vi "RomiSim_WriteSensors.vi"(10 "Diff Drive Train Sim":T8 {"m_Motor"."Jr_KgM2" format="%13.5p"; "m_Motor"."L_H" format="%13.5p"; "m_Motor"."Kt_NMPerAmp" format="%13.5p"; "m_Motor"."KvINV_RadPerSecPerVolt" format="%13.5p"; "m_Motor"."R_Ohms" format="%13.5p"; "m_Motor"."FreeSpeed_RadPerSec" format="%13.5p"; "m_Motor"."FreeCurrent_Amps" format="%13.5p"; "m_Motor"."StallCurrent_Amps" format="%13.5p"; "m_Motor"."StallTorque_NM" format="%13.5p"; "m_Motor"."nominalVoltage_Volts" format="%13.5p"}, 11 "Counts/Feet":dbl) -> (0 "Right Speed Ft/Sec":dbl, 1 "Right Encoder":T6, 2 "Left Speed Ft/Sec":dbl, 3 "Left Encoder":T6, 4 "Robot Pose":T3 {"ROTATION"."SIN" format="%13.4f"; "ROTATION"."COS" format="%13.4f"; "ROTATION"."VALUE" format="%13.4f"; "TRANSLATION"."Y" format="%14.3f"; "TRANSLATION"."X" format="%14.3f"}, 5 "Gyro Deg":dbl, 7 "Gyro":T1)   [LabVIEW 2019]
uses:
  <vilib>/Rock Robotics/WPI/ThirdParty/JAS_Junk/TrajLib/TypeDef/DIFF_DRIVE_TRAIN_SIM.ctl
  <vilib>/Rock Robotics/WPI/ThirdParty/JAS_Junk/TrajLib/TypeDef/LINEAR_SYSTEM.ctl
  <vilib>/Analysis/Matrix/Datatypes/RealMatrix.ctl
  <vilib>/Rock Robotics/WPI/ThirdParty/JAS_Junk/TrajLib/TypeDef/DCMOTOR.CTL
  <vilib>/Rock Robotics/WPI/Simulation/Protocol/Devices/Encoder/Encoder proto.ctl
  <vilib>/Rock Robotics/WPI/Simulation/Protocol/Devices/Encoder/Encoder data protoo.ctl
  <vilib>/Rock Robotics/WPI/ThirdParty/JAS_Junk/TrajLib/TypeDef/POSE2D.ctl
  <vilib>/Rock Robotics/WPI/ThirdParty/JAS_Junk/TrajLib/TypeDef/TRANSLATION2D.ctl
  <vilib>/Rock Robotics/WPI/ThirdParty/JAS_Junk/TrajLib/TypeDef/ROTATION2D.ctl
  <vilib>/Rock Robotics/WPI/Simulation/Protocol/Devices/Gyro/Gyro proto.ctl
  <vilib>/Rock Robotics/WPI/Simulation/Protocol/Devices/Gyro/Gyro Data proto.ctl
  <vilib>/Rock Robotics/WPI/Simulation/Protocol/Devices/Encoder/Encoder Update Ops.ctl
  <vilib>/Rock Robotics/SystemInterfaces/Encoder/FPGA_EncoderIdx.ctl
  <vilib>/Rock Robotics/WPI/Simulation/Protocol/Devices/Gyro/Gyro Update Ops.ctl
  <vilib>/Rock Robotics/WPI/ThirdParty/JAS_Junk/TrajLib/Trajectory_Library.lvlib
  <vilib>/Analysis/Matrix/NI_Matrix.lvlib
panel:
  # "<States, 1>"
  # "<Outputs, 1>"
  # "<Inputs, 1>"
  # "<Outputs, 1>"
  # "<States,States>"
  # "<States,Inputs>"
  # "<Outputs,States>"
  # "<Outputs,Inputs>"
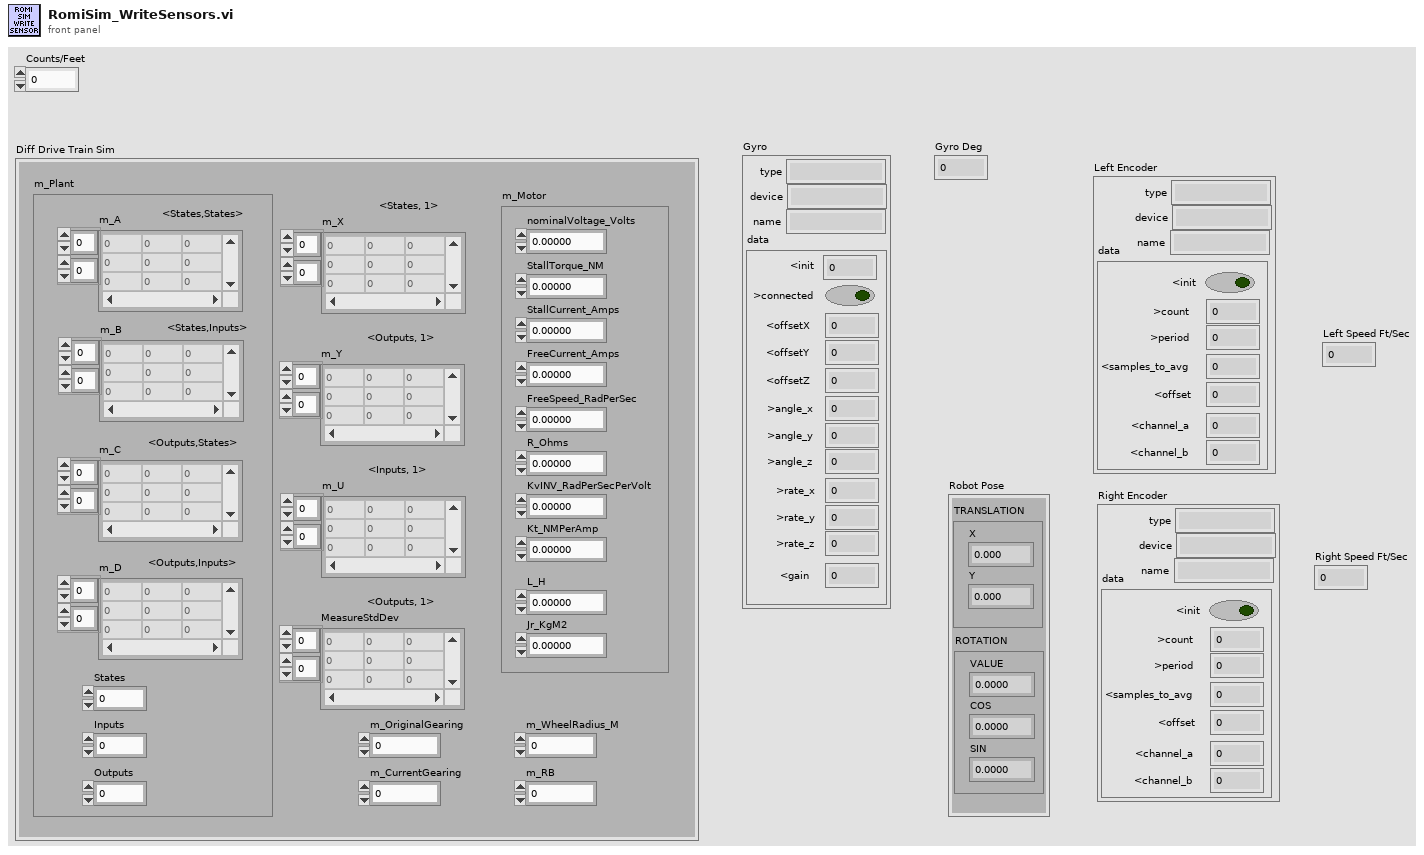
[diagram p1: front panel]
types:
  T1 = typedef "Gyro proto.ctl" = cluster{"type":string, "device":string, "name":string, "data":T2}
  T2 = typedef "Gyro Data proto.ctl" = cluster{"<init":i32, ">connected":bool, "<offsetX":dbl, "<offsetY":dbl, "<offsetZ":dbl, ">angle_x":dbl, ">angle_y":dbl, ">angle_z":dbl, ">rate_x":dbl, ">rate_y":dbl, ">rate_z":dbl, "<gain":dbl}
  T3 = typedef "Trajectory_Library.lvlib/POSE2D.ctl" = cluster{"TRANSLATION":T4, "ROTATION":T5}
  T4 = typedef "Trajectory_Library.lvlib/TRANSLATION2D.ctl" = cluster{"X":dbl, "Y":dbl}
  T5 = typedef "Trajectory_Library.lvlib/ROTATION2D.ctl" = cluster{"VALUE":dbl, "COS":dbl, "SIN":dbl}
  T6 = typedef "Encoder proto.ctl" = cluster{"type":string, "device":string, "name":string, "data":T7}
  T7 = typedef "Encoder data protoo.ctl" = cluster{"<init":bool, ">count":dbl, ">period":dbl, "<samples_to_avg":i32, "<offset":dbl, "<channel_a":i32, "<channel_b":i32}
  T8 = typedef "Trajectory_Library.lvlib/DIFF_DRIVE_TRAIN_SIM.ctl" = cluster{"m_Plant":T9, "m_X":T10, "m_Y":T10, "m_U":T10, "MeasureStdDev":T10, "m_Motor":T11, "m_OriginalGearing":dbl, "m_CurrentGearing":dbl, "m_WheelRadius_M":dbl, "m_RB":dbl}
  T9 = typedef "Trajectory_Library.lvlib/LINEAR_SYSTEM.ctl" = cluster{"m_A":T10, "m_B":T10, "m_C":T10, "m_D":T10, "States":i32, "Inputs":i32, "Outputs":i32}
  T10 = typedef "NI_Matrix.lvlib/RealMatrix.ctl" = dbl[][]
  T11 = typedef "Trajectory_Library.lvlib/DCMOTOR.CTL" = cluster{"nominalVoltage_Volts":dbl, "StallTorque_NM":dbl, "StallCurrent_Amps":dbl, "FreeCurrent_Amps":dbl, "FreeSpeed_RadPerSec":dbl, "R_Ohms":dbl, "KvINV_RadPerSecPerVolt":dbl, "Kt_NMPerAmp":dbl, "L_H":dbl, "Jr_KgM2":dbl}
  T12 = typedef "Gyro Update Ops.ctl" = enum16{"get", "delete", "JSON update", "set  name", "transmit initial", "reset", "set init", "set offsetX", "set offsetY", "set offsetZ", "set gain", "set angle X", "set angle Y", "set angle Z", "set rate X", "set rate Y", "set rate Z"}
  T13 = typedef "Encoder Update Ops.ctl" = enum16{"set init", "set count", "set period", "set reset", "set samples_to_avg", "get", "delete", "JSON update", "set name", "transmit initial", "reset", "set channel_a", "set channel_b"}
  T14 = typedef "FPGA_EncoderIdx.ctl" = enum8{"Enc 0", "Enc 1", "Enc 2", "Enc 3", "Enc 4", "Enc 5", "Enc 6", "Enc 7", "Invalid"}
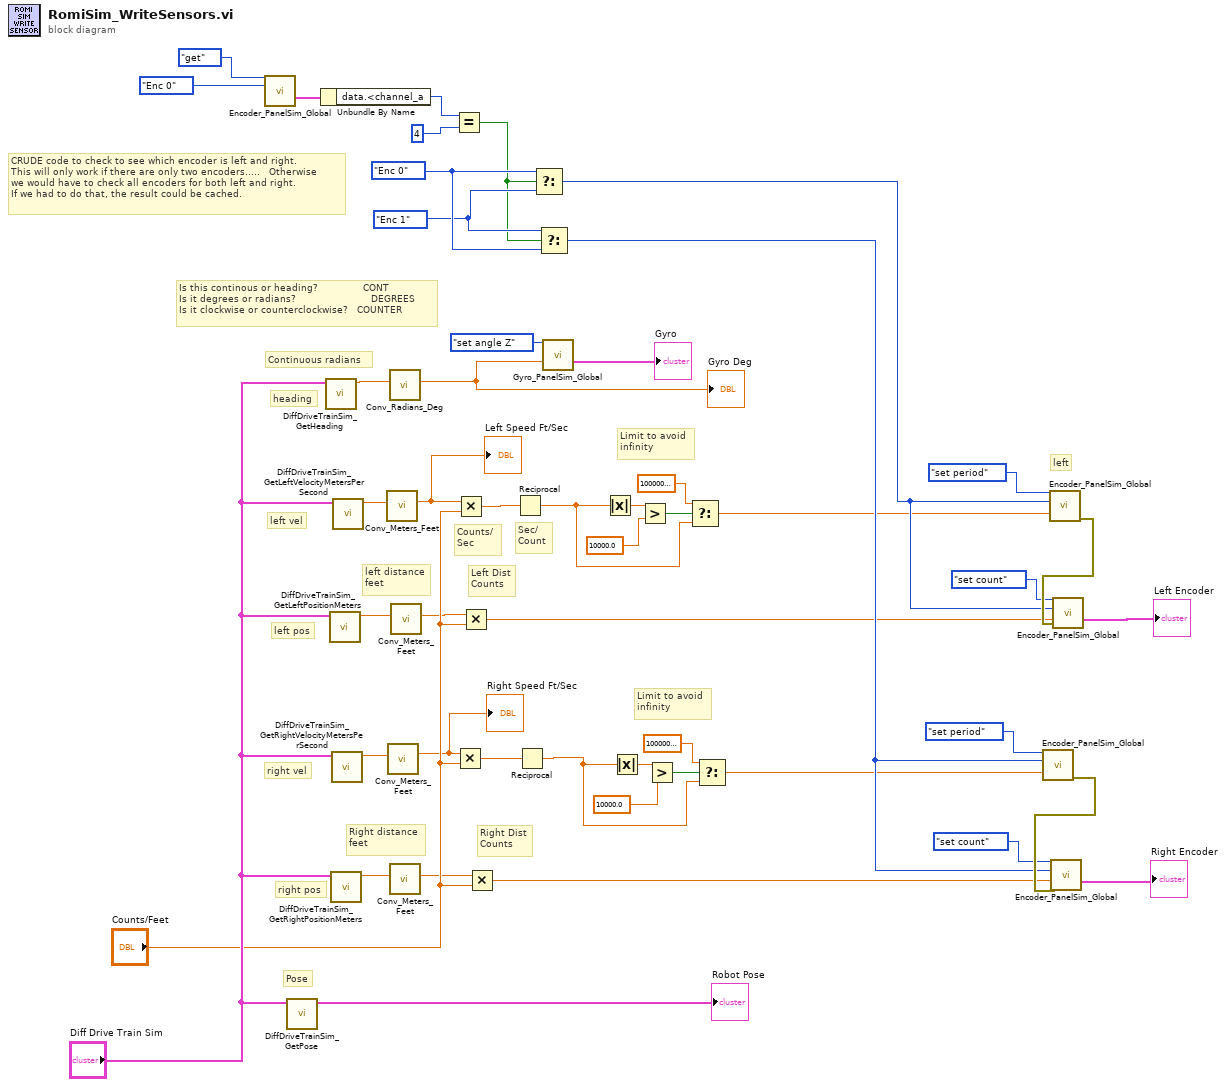
[diagram p0: block diagram]
diagram:
  w33 = FPGA_EncoderIdx."Enc 1" ("EncoderIndex")
  w34 = FPGA_EncoderIdx."Enc 0" ("EncoderIndex")
  # "Limit to avoid\ninfinity"
  # "left"
  # "CRUDE code to check to see which encoder is left and right.\nThis will only work if there are only two encoders.....   Otherwise\nwe would have to check all encoders for both left and right.\nIf we had to do that, the result could be cached."
  # "Right Dist\nCounts"
  # "Left Dist\nCounts"
  # "Is this continous or heading?               CONT\nIs it degrees or radians?                         DEGREES\nIs it clockwise or counterclockwise?   COUNTER"
  # "Sec/\nCount"
  # "Limit to avoid\ninfinity"
  # "Counts/\nSec"
  # "Continuous radians"
  # "Right distance\nfeet"
  # "left distance\nfeet"
  # "heading"
  # "left pos"
  # "right pos"
  # "right vel"
  # "left vel"
  # "Pose"
  n1 = call <vilib>:"Encoder_PanelSim_Global.vi"("menu"=Encoder_Update_Ops."get", "EncoderIndex"=FPGA_EncoderIdx."Enc 0") -> ("Encoder new"=w29:T6)  [unwired: 12 in, 1 out]
  n2 = call <vilib>:"DiffDriveTrainSim_GetPose.vi"("DiffDriveTrainSim"="Diff Drive Train Sim") -> ("Pose"=→"Robot Pose":T3)  [unwired: 10 in]
  n3 = Unbundle By Name(w29) -> ("data.<channel_a"=w30:i32)
  n4 = call <vilib>:"DiffDriveTrainSim_GetHeading.vi"("DiffDriveTrainSim"="Diff Drive Train Sim") -> ("Heading"=w46:dbl)  [unwired: 10 in]
  n5 = call <vilib>:"DiffDriveTrainSim_GetLeftPositionMeters.vi"("DiffDriveTrainSim"="Diff Drive Train Sim") -> ("LeftPosition_Meters"=w16:dbl)  [unwired: 10 in]
  n6 = call <vilib>:"DiffDriveTrainSim_GetRightPositionMeters.vi"("DiffDriveTrainSim"="Diff Drive Train Sim") -> ("RightPosition_Meters"=w13:dbl)  [unwired: 10 in]
  n7 = call <vilib>:"DiffDriveTrainSim_GetRightVelocityMetersPerSecond.vi"("DiffDriveTrainSim"="Diff Drive Train Sim") -> ("RightVel_M_Per_Sec"=w14:dbl)  [unwired: 10 in]
  n8 = call <vilib>:"DiffDriveTrainSim_GetLeftVelocityMetersPerSecond.vi"("DiffDriveTrainSim"="Diff Drive Train Sim") -> ("LeftVelocity_M_Per_Sec"=w15:dbl)  [unwired: 10 in]
  n9 = call <vilib>:"Conv_Meters_Feet.vi"("Meters"=w15) -> ("Feet"=w37:dbl)  [unwired: 10 in]
  "Left Speed Ft/Sec" <- w37
  n10 = call <vilib>:"Conv_Meters_Feet.vi"("Meters"=w14) -> ("Feet"=w17:dbl)  [unwired: 10 in]
  "Right Speed Ft/Sec" <- w17
  n11 = call <vilib>:"Conv_Radians_Deg.vi"("Radians"=w46) -> ("Degrees"=w47:dbl)  [unwired: 10 in]
  "Gyro Deg" <- w47
  n12 = call <vilib>:"Conv_Meters_Feet.vi"("Meters"=w13) -> ("Feet"=w22:dbl)  [unwired: 10 in]
  n13 = call <vilib>:"Conv_Meters_Feet.vi"("Meters"=w16) -> ("Feet"=w23:dbl)  [unwired: 10 in]
  n14 = Equal?(x=w30, y=4) -> (x = y?=w32:bool)
  n15 = Multiply(x=w17, y="Counts/Feet") -> (x*y=w18:dbl)
  n16 = Multiply(x=w37, y="Counts/Feet") -> (x*y=w19:dbl)
  n17 = Multiply(x=w23, y="Counts/Feet") -> (x*y=w25:dbl)
  n18 = Multiply(x=w22, y="Counts/Feet") -> (x*y=w26:dbl)
  n19 = Reciprocal(x=w19) -> (1/x=w21:dbl)
  n20 = Reciprocal(x=w18) -> (1/x=w20:dbl)
  n21 = Select(t=w34, s=w32, f=w33) -> (s? t:f=w35:T14)
  n22 = Select(t=w33, s=w32, f=w34) -> (s? t:f=w36:T14)
  n23 = call <vilib>:"Gyro_PanelSim_Global.vi"("Menu"=Gyro_Update_Ops."set angle Z", "Numeric Value"=w47) -> ("Value out"=→"Gyro":T1)  [unwired: 12 in, 1 out]
  n24 = Absolute Value(x=w21) -> (abs(x)=w2:dbl)
  n25 = Absolute Value(x=w20) -> (abs(x)=w6:dbl)
  n26 = Greater?(x=w2, y=10000.0) -> (0:w4:bool)
  n27 = Greater?(x=w6, y=10000.0) -> (0:w8:bool)
  n28 = Select(t=100000000000000.0, s=w4, f=w21) -> (s? t:f=w10:dbl)
  n29 = Select(t=100000000000000.0, s=w8, f=w20) -> (s? t:f=w11:dbl)
  n30 = call <vilib>:"Encoder_PanelSim_Global.vi"("menu"=Encoder_Update_Ops."set period", "EncoderIndex"=w36, "Numeric Value"=w11) -> ("error out"=w44:errorcluster)  [unwired: 11 in, 1 out]
  n31 = call <vilib>:"Encoder_PanelSim_Global.vi"("menu"=Encoder_Update_Ops."set period", "EncoderIndex"=w35, "Numeric Value"=w10) -> ("error out"=w42:errorcluster)  [unwired: 11 in, 1 out]
  n32 = call <vilib>:"Encoder_PanelSim_Global.vi"("menu"=Encoder_Update_Ops."set count", "EncoderIndex"=w36, "Numeric Value"=w26, "error in (no error)"=w44) -> ("Encoder new"=→"Right Encoder":T6)  [unwired: 10 in, 1 out]
  n33 = call <vilib>:"Encoder_PanelSim_Global.vi"("menu"=Encoder_Update_Ops."set count", "EncoderIndex"=w35, "Numeric Value"=w25, "error in (no error)"=w42) -> ("Encoder new"=→"Left Encoder":T6)  [unwired: 10 in, 1 out]
